vi "Auto Analysis.vi"(8 "error in (no error)":errorcluster, 11 "Yokogawa AQ6370D in":refnum<class "Yokogawa AQ6370D.lvclass">) -> (0 "error out":errorcluster, 2 "Analysis Data":T1, 3 "Yokogawa AQ6370D out":refnum<class "Yokogawa AQ6370D.lvclass">)   [LabVIEW 2018, in "Yokogawa AQ6370D.lvlib" / "Yokogawa AQ6370D.lvclass"]
uses:
  Yokogawa AQ6370D.lvclass
  PPLs/Optical Spectrum Analyzer/Parent/OSA.lvlibp/Custom Controls/Analysis Data.ctl
  Yokogawa AQ6370D.lvclass/Yokogawa AQ6370D.ctl
  PPLs/Optical Spectrum Analyzer/Parent/OSA.lvlibp/Optical Spectrum Analyzer.lvclass
  C:/Projects/LabVIEW/PPLs/Optical Spectrum Analyzer/Parent/OSA.lvlibp/Optical Spectrum Analyzer.lvclass
panel:
  out "Total Power":dbl format="%.4f"
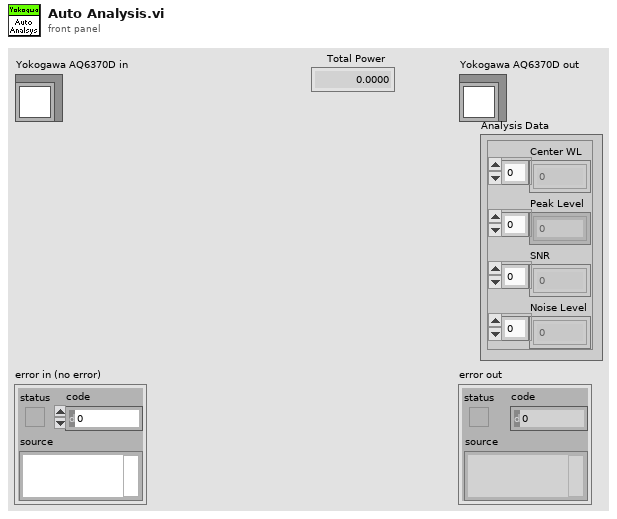
[diagram p1: front panel]
types:
  T1 = typedef "OSA.lvlibp/Optical Spectrum Analyzer.lvclass/Analysis Data.ctl" = cluster{"Center WL":dbl[], "Peak Level":dbl[], "SNR":dbl[], "Noise Level":dbl[]}
  T2 = cluster{"Channel Detection":cluster{"Threshold Level":dbl, "Mode Diff":dbl}, "Interpolation":cluster{"Noise BW":dbl, "Noise Config":enum16{"Auto Fix", "Manual Fix", "Auto Center", "Manual Center"}, "Fitting Config":enum16{"Linear", "Gauss", "Lorenz", "3rd Poly", "4th Poly", "5th Poly"}, "Noise Area (nm)":dbl, "Mask Area (nm)":dbl}}
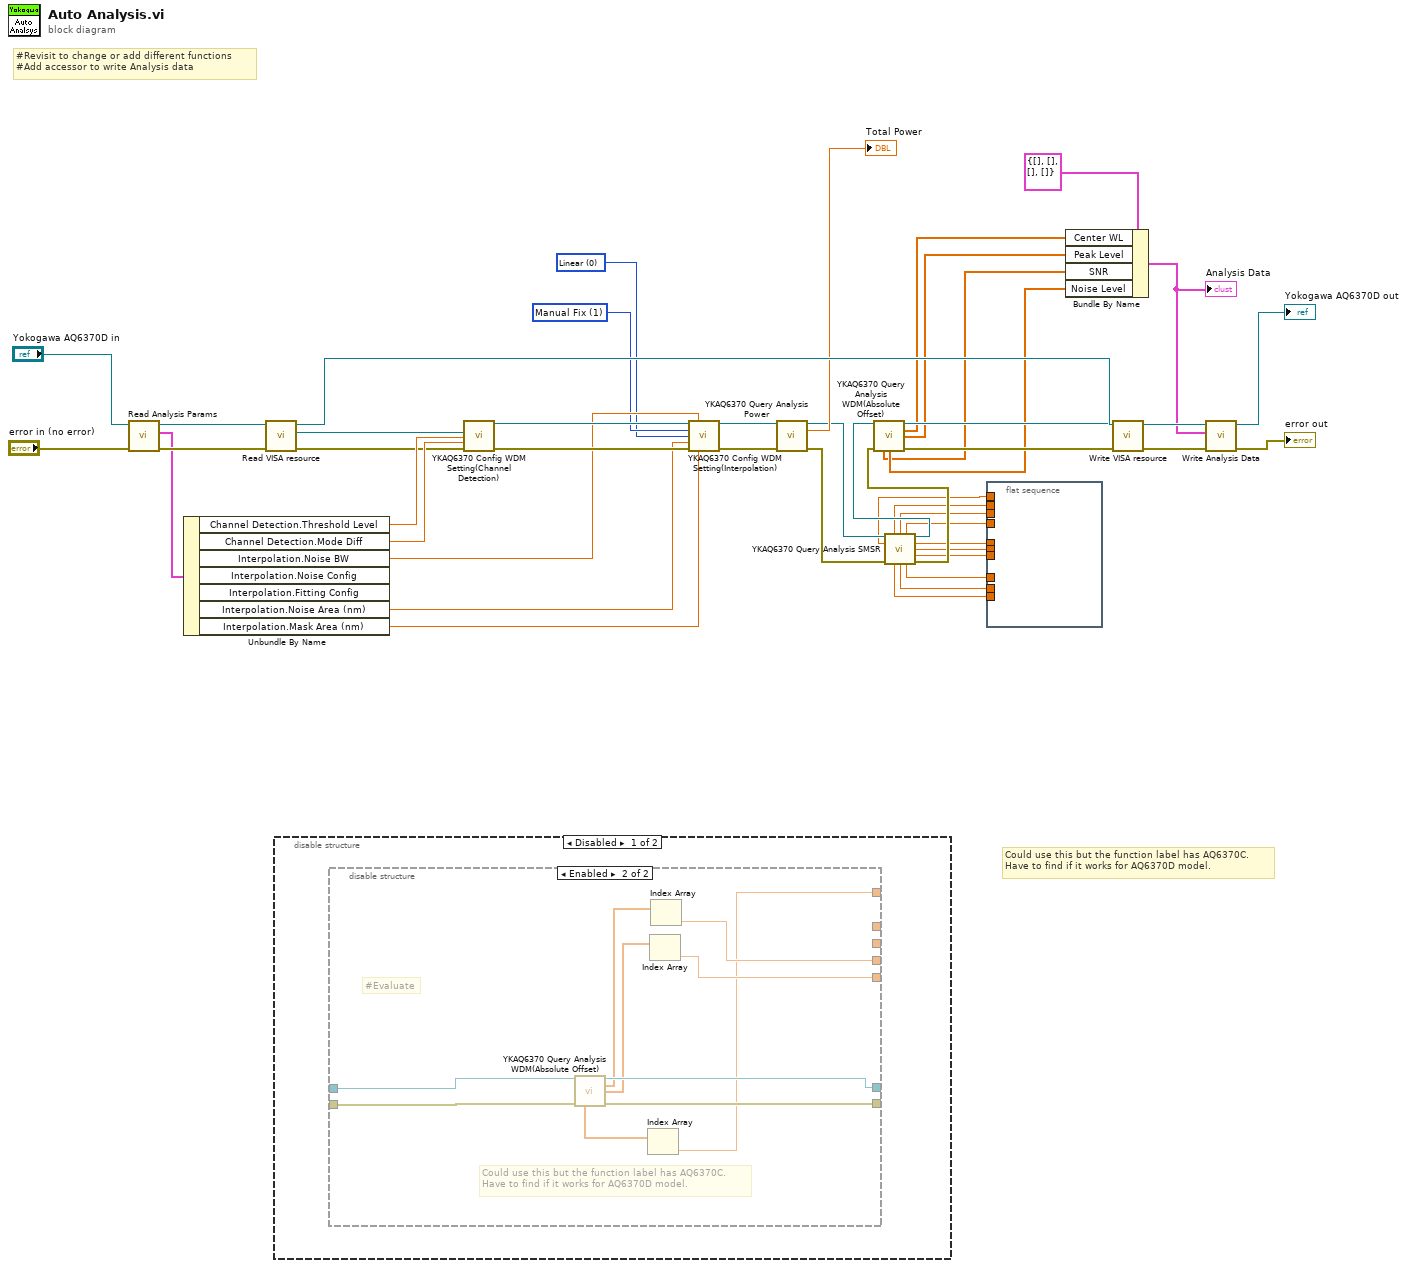
[diagram p0: block diagram]
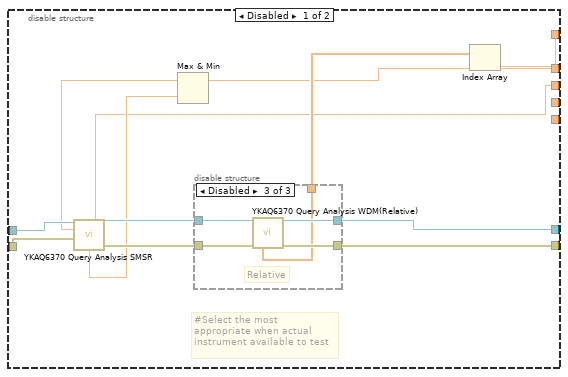
[diagram p2: hidden frame]
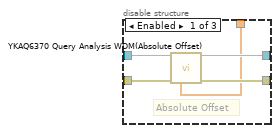
[diagram p3: hidden frame]
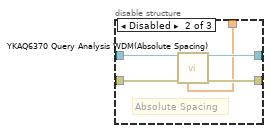
[diagram p4: hidden frame]
diagram:
  w24 = u16 0 items=["Linear", "Gauss", "Lorenz", "3rd Poly", "4th Poly", "5th Poly"] ("Fitting Algo (0: linear)")
  w25 = u16 1 items=["Auto Fix", "Manual Fix", "Auto Center", "Manual Center", "PIT"] ("Noise Algo (0: Auto Fix)")
  # "Could use this but the function label has AQ6370C.\nHave to find if it works for AQ6370D model."
  # "#Revisit to change or add different functions\n#Add accessor to write Analysis data"
  n1 = call "Read Analysis Params.vi"("error in (no error)"="error in (no error)", "Optical Spectrum Analyzer in"="Yokogawa AQ6370D in") -> ("error out"=w34:errorcluster, "Analysis Params"=w33:T2, "Optical Spectrum Analyzer out"=w35:refnum<class "Yokogawa AQ6370D.lvclass">)  [unwired: 7 in]
  n2 = Unbundle By Name(w33) -> ("Channel Detection.Threshold Level"=w31:dbl, "Channel Detection.Mode Diff"=w30:dbl, "Interpolation.Noise BW"=w26:dbl, "Interpolation.Noise Area (nm)"=w23:dbl, "Interpolation.Mask Area (nm)"=w22:dbl)  [unwired: 2 out]
  n3 = call "Read VISA resource.vi"("error in (no error)"=w34, "Yokogawa AQ6370D in"=w35) -> ("error out"=w29:errorcluster, "VISA resource"=w32:refnum<visa-resource-name>, "Yokogawa AQ6370D out"=w45:refnum<class "Yokogawa AQ6370D.lvclass">)  [unwired: 7 in]
  n4 = disable-structure shown="Disabled" {
    frame Disabled {
      n5 = disable-structure shown="Enabled" {
        disable-tunnel: _ -> [w58 w82]
        disable-tunnel: _ -> [w57 w83]
        disable-tunnel: [w54 w81] -> _
        disable-tunnel: [w53 w80] -> _
        disable-tunnel: [w49 w74] -> _
        disable-tunnel: [w47 _] -> _
        disable-tunnel: [w48 _] -> _
        disable-tunnel: [_ w78] -> _
        disable-tunnel: [_ w76] -> _
        frame Disabled {
          # "#Select the most \nappropriate when actual \ninstrument available to test"
          n6 = call <instrlib>:"YKAQ6370 Query Analysis SMSR.vi"("VISA resource name"=w57, "error in (no error)"=w58) -> ("Peak WL"=w48:dbl, "VISA resource name out"=w55:refnum<visa-resource-name>, "Delta Level(R)"=w51:dbl, "Delta Level"=w52:dbl, "error out"=w56:errorcluster)  [unwired: 2 in, 7 out]
          n7 = Max & Min(x=w51, y=w52) -> (max(x,y)=w47:dbl)  [unwired: 1 out]
          n8 = disable-structure shown="Disabled" {
            disable-tunnel: w56 -> [w63 w67 w70]
            disable-tunnel: w55 -> [w62 w68 w73]
            disable-tunnel: [w61 w65 w71] -> w54
            disable-tunnel: [w60 w66 w72] -> w53
            disable-tunnel: [w59 w64 w69] -> w50
            frame Enabled {
              # "Absolute Offset"
              n9 = call <instrlib>:"YKAQ6370 Query Analysis WDM(Absolute Offset).vi"("VISA resource name"=w62, "error in (no error)"=w63) -> ("VISA resource name out"=w60:refnum<visa-resource-name>, "SNR"=w59:dbl[], "error out"=w61:errorcluster)  [unwired: 5 in, 6 out]
            }
            frame Disabled {
              # "Absolute Spacing"
              n10 = call <instrlib>:"YKAQ6370 Query Analysis WDM(Absolute Spacing).vi"("VISA resource name"=w68, "error in (no error)"=w67) -> ("VISA resource name out"=w66:refnum<visa-resource-name>, "SNR"=w64:dbl[], "error out"=w65:errorcluster)  [unwired: 5 in, 6 out]
            }
            frame Disabled {
              # "Relative"
              n11 = call <instrlib>:"YKAQ6370 Query Analysis WDM(Relative).vi"("VISA resource name"=w73, "error in (no error)"=w70) -> ("VISA resource name out"=w72:refnum<visa-resource-name>, "SNR"=w69:dbl[], "error out"=w71:errorcluster)  [unwired: 5 in, 6 out]
            }
          }
          n12 = Index Array(array=w50) -> (element=w49:dbl)  [unwired: 1 in]
        }
        frame Enabled {
          # "#Evaluate"
          # "Could use this but the function label has AQ6370C.\nHave to find if it works for AQ6370D model."
          n13 = call <instrlib>:"YKAQ6370 Query Analysis WDM(Absolute Offset).vi"("VISA resource name"=w83, "error in (no error)"=w82) -> ("VISA resource name out"=w80:refnum<visa-resource-name>, "Center WL"=w79:dbl[], "Peak Level"=w77:dbl[], "SNR"=w75:dbl[], "error out"=w81:errorcluster)  [unwired: 5 in, 4 out]
          n14 = Index Array(array=w75) -> (element=w74:dbl)  [unwired: 1 in]
          n15 = Index Array(array=w77) -> (element=w76:dbl)  [unwired: 1 in]
          n16 = Index Array(array=w79) -> (element=w78:dbl)  [unwired: 1 in]
        }
      }
    }
    frame Enabled {
    }
  }
  n17 = call <instrlib>:"YKAQ6370 Config WDM Setting(Channel Detection).vi"("VISA resource name"=w32, "Thresh Level (20.0)"=w31, "Mode Diff (3.00)"=w30, "error in (no error)"=w29) -> ("VISA resource name out"=w28:refnum<visa-resource-name>, "error out"=w27:errorcluster)  [unwired: 10 in]
  n18 = call <instrlib>:"YKAQ6370 Config WDM Setting(Interpolation).vi"("VISA resource name"=w28, "Noise Bandwidth (0.10)"=w26, "Noise Algo (0: Auto Fix)"=w25, "Fitting Algo (0: linear)"=w24, "Noise Area (0.40)"=w23, "error in (no error)"=w27, "Mask Area (0.20)"=w22) -> ("VISA resource name out"=w2:refnum<visa-resource-name>, "error out"=w1:errorcluster)  [unwired: 7 in]
  n19 = call <instrlib>:"YKAQ6370 Query Analysis Power.vi"("VISA resource name"=w2, "error in (no error)"=w1) -> ("VISA resource name out"=w16:refnum<visa-resource-name>, "Total Power"=→"Total Power":dbl, "error out"=w15:errorcluster)  [unwired: 11 in]
  n20 = call <instrlib>:"YKAQ6370 Query Analysis SMSR.vi"("VISA resource name"=w16, "error in (no error)"=w15) -> ("2nd Peak Level(R)"=w11:dbl, "2nd Peak WL(R)"=w10:dbl, "Peak WL"=w9:dbl, "VISA resource name out"=w14:refnum<visa-resource-name>, "Delta Level(R)"=w12:dbl, "Peak Level"=w8:dbl, "2nd Peak WL"=w7:dbl, "2nd Peak Level"=w6:dbl, "Delta WL(R)"=w3:dbl, "Delta Level"=w4:dbl, "Delta WL"=w5:dbl, "error out"=w13:errorcluster)  [unwired: 2 in]
  n21 = call <instrlib>:"YKAQ6370 Query Analysis WDM(Absolute Offset).vi"("VISA resource name"=w14, "error in (no error)"=w13) -> ("VISA resource name out"=w44:refnum<visa-resource-name>, "Center WL"=w21:dbl[], "Peak Level"=w20:dbl[], "SNR"=w18:dbl[], "Noise"=w19:dbl[], "error out"=w46:errorcluster)  [unwired: 5 in, 3 out]
  n22 = flat-sequence {
    tunnel: w12 -> [_]
    tunnel: w11 -> [_]
    tunnel: w10 -> [_]
    tunnel: w9 -> [_]
    tunnel: w8 -> [_]
    tunnel: w7 -> [_]
    tunnel: w6 -> [_]
    tunnel: w5 -> [_]
    tunnel: w4 -> [_]
    tunnel: w3 -> [_]
    frame #0 {
    }
  }
  n23 = Bundle By Name(cluster=T1 {"Center WL"=[], "Peak Level"=[], "SNR"=[], "Noise Level"=[]} ("Analysis Data"), "Center WL"=w21, "Peak Level"=w20, "SNR"=w18, "Noise Level"=w19) -> (w39:T1)
  "Analysis Data" <- w39
  n24 = call "Write VISA resource.vi"("error in (no error)"=w46, "VISA resource"=w44, "Yokogawa AQ6370D in"=w45) -> ("error out"=w42:errorcluster, "Yokogawa AQ6370D out"=w43:refnum<class "Yokogawa AQ6370D.lvclass">)  [unwired: 7 in]
  n25 = call "Write Analysis Data.vi"("error in (no error)"=w42, "Analysis Data"=w39, "Optical Spectrum Analyzer in"=w43) -> ("error out"=→"error out":errorcluster, "Optical Spectrum Analyzer out"=→"Yokogawa AQ6370D out":refnum<class "Yokogawa AQ6370D.lvclass">)  [unwired: 7 in]
